vi "DestroySelfReference.vi"(8 "error in (no error)":errorcluster, 11 "SMU.Keithley2600":refnum<class "SMU.Keithley2600.lvclass">) -> (0 "error out":errorcluster, 3 "SMU.Keithley2600 out":refnum<class "SMU.Keithley2600.lvclass">)   [LabVIEW 2017, in "SMU.Keithley2600.lvclass"]
doc: "JKI State Machine Objects (SMO) 1.0.0.5\nJKI - JKI\nCopyright (c) 2016, JKI"
uses:
  SMU.Keithley2600.lvclass
  SMU.Keithley2600.lvclass/SMU.Keithley2600.ctl
  SMU/SMU.lvclass
panel:
  # "For instructions on how to use the JKI State Machine Objects, examples and video tutorials, visit:\nhttp://jki.net/state-machine-objects/\n\nJKI State Machine Objects™\nhttp://jki.net/state-machine-objects/\nCopyright (C) 2005-2015, JKI <info@jki.net>\nALL RIGHTS RESERVED"
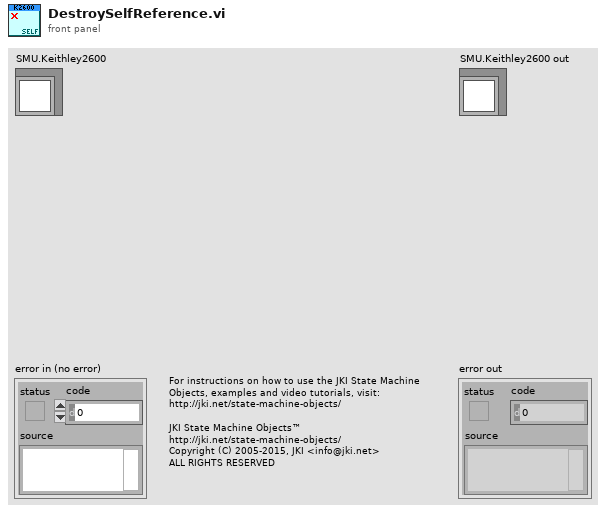
[diagram p1: front panel]
types:
  T1 = typedef "SMU.Keithley2600.lvclass/PrivateData--Ref.ctl" = refnum<data-value>
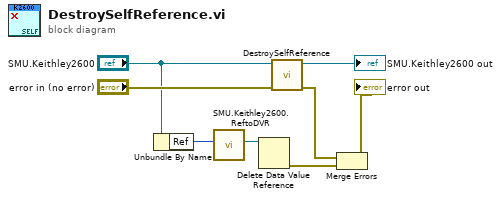
[diagram p0: block diagram]
diagram:
  n1 = Unbundle By Name("SMU.Keithley2600") -> ("Ref"=w2:u32)
  n2 = call "SMU.Keithley2600.ReftoDVR.vi"("Ref"=w2) -> ("Ref"=w1:T1)  [unwired: 10 in]
  n3 = Delete Data Value Reference(data value reference=w1) -> (error out=w5:errorcluster)  [unwired: 1 in, 1 out]
  n4 = call-parent "DestroySelfReference.vi"("error in (no error)"="error in (no error)", "SMU"="SMU.Keithley2600") -> ("error out"=w4:errorcluster, "SMU out"=→"SMU.Keithley2600 out":refnum<class "SMU.Keithley2600.lvclass">)  [unwired: 8 in]
  n5 = Merge Errors(w4, w5) -> (→"error out":errorcluster)
